vi "ProcessName.vi"() -> (1 "process name":string)   [LabVIEW 2017, in "TimerProcess.lvlib"]
uses:
  <vilib>/addons/TimerProcess/TimerProcess.lvlib
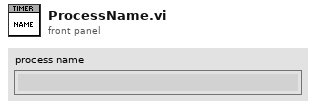
[diagram p1: front panel]
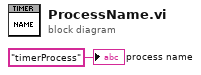
[diagram p0: block diagram]
diagram:
  "process name" <- "timerProcess" ("ProcessName")
